vi "ESP301_Set_Limit.vi"(8 "limit_l":dbl, 9 "limit_r":dbl, 10 "axisNumber":i32=1, 11 "COM_PORT":string="COM12") -> ()   [LabVIEW 2019]
uses:
  Newport.ESP301.CommandInterface
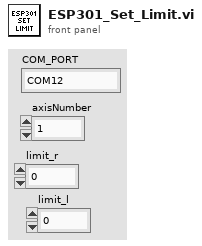
[diagram p1: front panel]
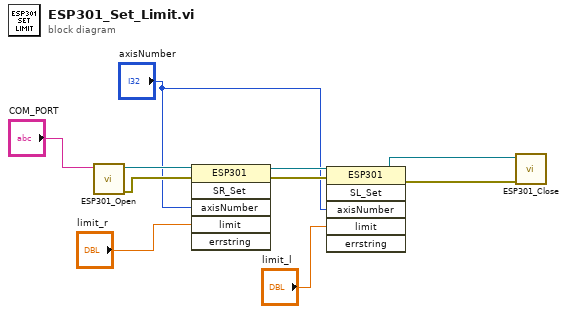
[diagram p0: block diagram]
diagram:
  n1 = call "ESP301_Open.vi"("strDeviceKey"="COM_PORT") -> ("sortie d'erreur"=w9:errorcluster, "référence en sortie"=w10:refnum<k24>)  [unwired: 9 in]
  n2 = invoke on="Nœud de méthode" class="ESP301" method="SR_Set"(reference=w10, error in=w9, "axisNumber"="axisNumber", "limit"="limit_r") -> (reference out=w7:refnum<k24>, error out=w6:errorcluster)  [unwired: 2 in, 4 out]
  n3 = invoke on="Nœud de méthode" class="ESP301" method="SL_Set"(reference=w7, error in=w6, "axisNumber"="axisNumber", "limit"="limit_l") -> (reference out=w5:refnum<k24>, error out=w4:errorcluster)  [unwired: 2 in, 4 out]
  n4 = call "ESP301_Close.vi"("entrée d'erreur (pas d'erreur)"=w4, "référence"=w5) -> ()  [unwired: 9 in, 1 out]
